vi "Fast Get All Channels FuncGlobal.vi"(5 "Action":enum16{"Open or Add", "Close Ref"}(ring), 8 "error in":errorcluster, 11 "Section Ref in":T1 format="%.0x") -> (0 "error out":errorcluster, 2 "Channel Refs":T1[](array[typedef]) format="%.0x", 3 "Section Ref out":T1 format="%.0x", 4 "Found":bool)   [LabVIEW 2011]
doc: "Returns an array of channel references for all the channels within the section specified by Section Ref in. This array includes references to both input and output channels.\n\nThis function performs a depth-first deep search for channels in the hierarchy."
uses:
  <vilib>/NI Veristand/Custom Device API/Custom Device Item Ref.ctl
  <vilib>/NI Veristand/Custom Device API/Custom Device API.lvlib
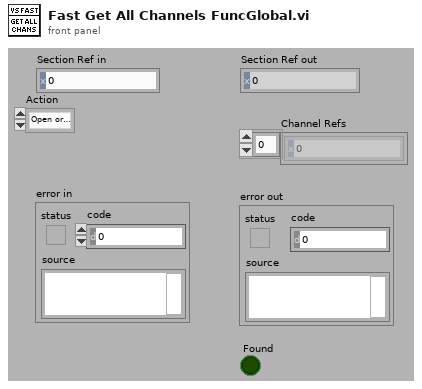
[diagram p1: front panel]
types:
  T1 = typedef "Custom Device API.lvlib/Custom Device Item Ref.ctl" = u64
  T2 = cluster{"Name":string, "Is Channel":bool, "GUID":string}
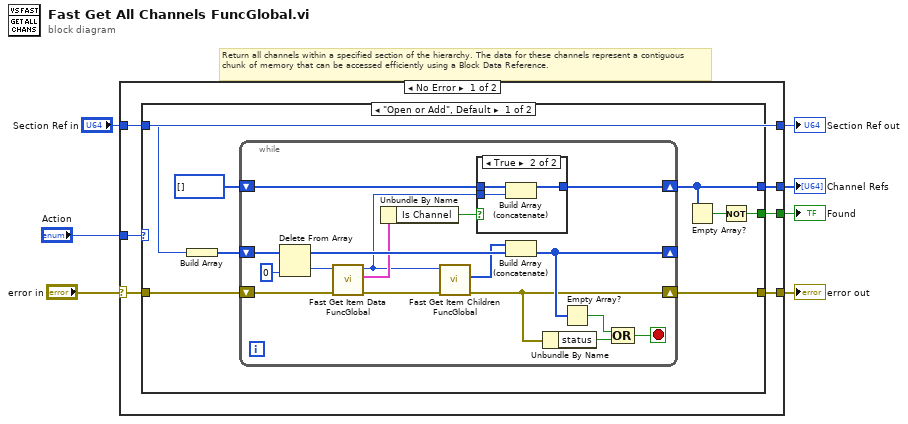
[diagram p0: block diagram]
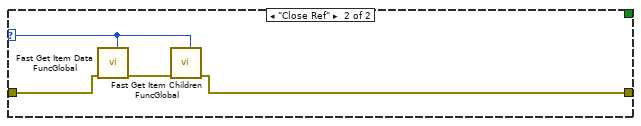
[diagram p3: hidden frame]
diagram:
  # "Return all channels within a specified section of the hierarchy. The data for these channels represent a contiguous chunk of memory that can be accessed efficiently using a Block Data Reference."
  n1 = case shown="No Error" "error in" {
    selector: "error in" -> [w10 w48]
    tunnel: "Section Ref in" -> [w9 w47]
    tunnel: [w13 w48] -> w6
    tunnel: [w12 _] -> w5
    tunnel: [w11 _] -> w4
    tunnel: [w9 w47] -> w2
    tunnel: "Action" -> [w8 _]
    frame No Error {
      n2 = case shown="\"Open or Add\", Default" w8 {
        selector: w8 -> [_ w44]
        tunnel: [w20 w43] -> w13
        tunnel: [w18 _] -> w12
        tunnel: [w16 _] -> w11
        tunnel: w10 -> [w15 w46]
        tunnel: w9 -> [w14 _]
        frame "Open or Add", Default {
          n3 = Build Array(w14) -> (w21:T1[])
          n4 = while {
            shift-right: [w24] -> w20
            shift-left: w15 -> [w27]
            shift-right: [w35] -> _
            shift-left: w21 -> [w38]
            shift-right: [w30] -> w18
            shift-left: T1[] [] ("appended array") -> [w31]
            stop <- w32 stop-if-true
            n5 = Delete From Array(array=w38, index=0) -> (deleted portion=w28:T1, array with subset deleted=w36:T1[])  [unwired: 1 in]
            n6 = call "Fast Get Item Data FuncGlobal.vi"("error in (no error)"=w27, "Item Ref in"=w28) -> ("error out"=w25:errorcluster, "Item Info"=w26:T2, "Item Ref out"=w22:T1)  [unwired: 6 in, 1 out]
            n7 = Unbundle By Name(w26) -> ("Is Channel"=w29:bool)
            n8 = call "Fast Get Item Children FuncGlobal.vi"("error in (no error)"=w25, "Item Ref in"=w22) -> ("error out"=w24:errorcluster, "Child Refs"=w23:T1[])  [unwired: 6 in, 2 out]
            n9 = case shown="True" w29 {
              tunnel: w31 -> [w39 w42]
              tunnel: [w39 w41] -> w30
              tunnel: w22 -> [_ w40]
              frame False {
              }
              frame True {
                n10 = Build Array (concatenate)(w42, w40) -> (w41:T1[])
              }
            }
            n11 = Build Array (concatenate)(w23, w36) -> (w35:T1[])
            n12 = Unbundle By Name(w24) -> ("status"=w34:bool)
            n13 = Empty Array?(array=w35) -> (empty?=w33:bool)
            n14 = Compound Arithmetic op=OR(w33, w34) -> (w32:bool)
          }
          n15 = Empty Array?(array=w18) -> (empty?=w17:bool)
          n16 = Not(x=w17) -> (.not. x?=w16:bool)
        }
        frame "Close Ref" {
          n17 = call "Fast Get Item Data FuncGlobal.vi"("Action"=w44, "error in (no error)"=w46) -> ("error out"=w45:errorcluster)  [unwired: 6 in, 3 out]
          n18 = call "Fast Get Item Children FuncGlobal.vi"("Action"=w44, "error in (no error)"=w45) -> ("error out"=w43:errorcluster)  [unwired: 6 in, 3 out]
        }
      }
    }
    frame Error {
    }
  }
  "Found" <- w4
  "error out" <- w6
  "Section Ref out" <- w2
  "Channel Refs" <- w5
